vi "read_config_file.vi"(8 "error in (no error)":errorcluster caption="错误输入（无错误）") -> (0 "error out":errorcluster caption="错误输出")   [LabVIEW 2015]
uses:
  globals/global_configuration_options.vi
  globals/global_device_tree_items.vi
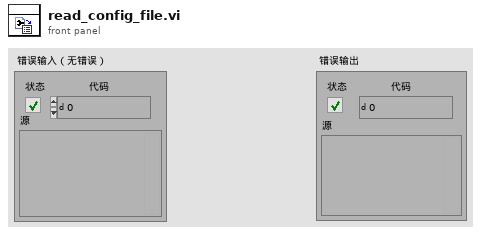
[diagram p1: front panel]
types:
  T1 = cluster{"Left Cell String":string, "Child Text":string[], "Child Tag":string, "Item Indent":i32, "Child Only?":bool, "Glyph Index":i32}[]
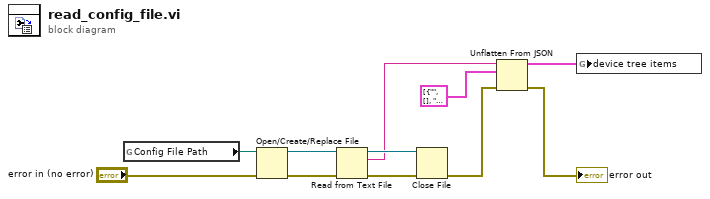
[diagram p0: block diagram]
diagram:
  n1 = global read "global_configuration_options.vi" "Config File Path"() -> (w11:path)
  n2 = Open/Create/Replace File(file path (use dialog)=w11, error in="error in (no error)") -> (refnum out=w9:refnum<file>, error out=w8:errorcluster)  [unwired: 4 in, 1 out]
  n3 = Read from Text File(file (use dialog)=w9, error in=w8) -> (refnum out=w7:refnum<file>, text=w5:string, error out=w6:errorcluster)  [unwired: 2 in, 1 out]
  n4 = Close File(refnum=w7, error in=w6) -> (error out=w4:errorcluster)  [unwired: 1 out]
  n5 = Unflatten From JSON(JSON string=w5, type and defaults=T1 [{"Left Cell String"="", "Child Text"=[], "Child Tag"="", "Item Indent"=0, "Child Only?"=FALSE, "Glyph Index"=1}, {"Left Cell String"="Mod1 (Slot1 NI 9239)", "Child Text"=[], "Child Tag"="Mod1", "Item Indent"=1, "Child Only?"=FALSE, "Glyph Index"=3}, {"Left Cell String"="FCXF-X-02-A01", "Child Text"=[], "Child Tag"="FCXF-X-02-A01", "Item Indent"=2, "Child Only?"=TRUE, "Glyph Index"=4}, {"Left Cell String"="FCXF-X-03-A01", "Child Text"=[], "Child Tag"="FCXF-X-03-A01", "Item Indent"=2, "Child Only?"=TRUE, "Glyph Index"=4}, {"Left Cell String"="FCXF-X-03-A02", "Child Text"=[], "Child Tag"="FCXF-X-03-A02", "Item Indent"=2, "Child Only?"=TRUE, "Glyph Index"=4}, {"Left Cell String"="FCXF-X-04-A01", "Child Text"=[], "Child Tag"="FCXF-X-04-A01", "Item Indent"=2, "Child Only?"=TRUE, "Glyph Index"=4}, {"Left Cell String"="Mod2 (Slot2 NI 9219)", "Child Text"=[], "Child Tag"="Mod2", "Item Indent"=1, "Child Only?"=FALSE, "Glyph Index"=3}, {"Left Cell String"="FCXF-X-02-S01", "Child Text"=[], "Child Tag"="FCXF-X-02-S01", "Item Indent"=2, "Child Only?"=TRUE, "Glyph Index"=4}, {"Left Cell String"="FCXF-X-02-S02", "Child Text"=[], "Child Tag"="FCXF-X-02-S02", "Item Indent"=2, "Child Only?"=TRUE, "Glyph Index"=4}, {"Left Cell String"="FCXF-X-02-S03", "Child Text"=[], "Child Tag"="FCXF-X-02-S03", "Item Indent"=2, "Child Only?"=TRUE, "Glyph Index"=4}, {"Left Cell String"="FCXF-X-02-S04", "Child Text"=[], "Child Tag"="FCXF-X-02-S04", "Item Indent"=2, "Child Only?"=TRUE, "Glyph Index"=4}, {"Left Cell String"="Mod4 (Slot4 NI 9219)", "Child Text"=[], "Child Tag"="Mod4", "Item Indent"=1, "Child Only?"=FALSE, "Glyph Index"=3}, {"Left Cell String"="FCXF-X-03-S01", "Child Text"=[], "Child Tag"="FCXF-X-03-S01", "Item Indent"=2, "Child Only?"=TRUE, "Glyph Index"=4}, {"Left Cell String"="FCXF-X-03-S02", "Child Text"=[], "Child Tag"="FCXF-X-03-S02", "Item Indent"=2, "Child Only?"=TRUE, "Glyph Index"=4}, {"Left Cell String"="FCXF-X-03-S03", "Child Text"=[], "Child Tag"="FCXF-X-03-S03", "Item Indent"=2, "Child Only?"=TRUE, "Glyph Index"=4}, {"Left Cell String"="FCXF-X-03-S04", "Child Text"=[], "Child Tag"="FCXF-X-03-S04", "Item Indent"=2, "Child Only?"=TRUE, "Glyph Index"=4}, {"Left Cell String"="Mod6 (Slot6 NI 9219)", "Child Text"=[], "Child Tag"="Mod6", "Item Indent"=1, "Child Only?"=FALSE, "Glyph Index"=3}, {"Left Cell String"="FCXF-X-03-S05", "Child Text"=[], "Child Tag"="FCXF-X-03-S05", "Item Indent"=2, "Child Only?"=TRUE, "Glyph Index"=4}, {"Left Cell String"="FCXF-X-03-S06", "Child Text"=[], "Child Tag"="FCXF-X-03-S06", "Item Indent"=2, "Child Only?"=TRUE, "Glyph Index"=4}, {"Left Cell String"="Mod8 (Slot8 NI 9219)", "Child Text"=[], "Child Tag"="Mod8", "Item Indent"=1, "Child Only?"=FALSE, "Glyph Index"=3}, {"Left Cell String"="FCXF-X-04-S01", "Child Text"=[], "Child Tag"="FCXF-X-04-S01", "Item Indent"=2, "Child Only?"=TRUE, "Glyph Index"=4}, {"Left Cell String"="FCXF-X-04-S02", "Child Text"=[], "Child Tag"="FCXF-X-04-S02", "Item Indent"=2, "Child Only?"=TRUE, "Glyph Index"=4}, {"Left Cell String"="FCXF-X-04-S03", "Child Text"=[], "Child Tag"="FCXF-X-04-S03", "Item Indent"=2, "Child Only?"=TRUE, "Glyph Index"=4}, {"Left Cell String"="FCXF-X-04-S04", "Child Text"=[], "Child Tag"="FCXF-X-04-S04", "Item Indent"=2, "Child Only?"=TRUE, "Glyph Index"=4}, {"Left Cell String"="Mod9 (USB1 ICPCON 7005)", "Child Text"=[], "Child Tag"="Mod9", "Item Indent"=1, "Child Only?"=FALSE, "Glyph Index"=3}, {"Left Cell String"="FCXF-X-02-T01", "Child Text"=[], "Child Tag"="FCXF-X-02-T01", "Item Indent"=2, "Child Only?"=TRUE, "Glyph Index"=4}, {"Left Cell String"="FCXF-X-02-T02", "Child Text"=[], "Child Tag"="FCXF-X-02-T02", "Item Indent"=2, "Child Only?"=TRUE, "Glyph Index"=4}, {"Left Cell String"="FCXF-X-02-T03", "Child Text"=[], "Child Tag"="FCXF-X-02-T03", "Item Indent"=2, "Child Only?"=TRUE, "Glyph Index"=4}, {"Left Cell String"="FCXF-X-02-T04", "Child Text"=[], "Child Tag"="FCXF-X-02-T04", "Item Indent"=2, "Child Only?"=TRUE, "Glyph Index"=4}, {"Left Cell String"="FCXF-X-03-T01", "Child Text"=[], "Child Tag"="FCXF-X-03-T01", "Item Indent"=2, "Child Only?"=TRUE, "Glyph Index"=4}, {"Left Cell String"="FCXF-X-03-T02", "Child Text"=[], "Child Tag"="FCXF-X-03-T02", "Item Indent"=2, "Child Only?"=TRUE, "Glyph Index"=4}, {"Left Cell String"="FCXF-X-03-T03", "Child Text"=[], "Child Tag"="FCXF-X-03-T03", "Item Indent"=2, "Child Only?"=TRUE, "Glyph Index"=4}, {"Left Cell String"="Mod10 (USB1 ICPCON 7005)", "Child Text"=[], "Child Tag"="Mod10", "Item Indent"=1, "Child Only?"=FALSE, "Glyph Index"=3}, {"Left Cell String"="FCXF-X-03-T04", "Child Text"=[], "Child Tag"="FCXF-X-03-T04", "Item Indent"=2, "Child Only?"=TRUE, "Glyph Index"=4}, {"Left Cell String"="FCXF-X-03-T05", "Child Text"=[], "Child Tag"="FCXF-X-03-T05", "Item Indent"=2, "Child Only?"=TRUE, "Glyph Index"=4}, {"Left Cell String"="FCXF-X-03-T06", "Child Text"=[], "Child Tag"="FCXF-X-03-T06", "Item Indent"=2, "Child Only?"=TRUE, "Glyph Index"=4}, {"Left Cell String"="FCXF-X-04-T01", "Child Text"=[], "Child Tag"="FCXF-X-04-T01", "Item Indent"=2, "Child Only?"=TRUE, "Glyph Index"=4}, {"Left Cell String"="FCXF-X-04-T02", "Child Text"=[], "Child Tag"="FCXF-X-04-T02", "Item Indent"=2, "Child Only?"=TRUE, "Glyph Index"=4}, {"Left Cell String"="FCXF-X-04-T03", "Child Text"=[], "Child Tag"="FCXF-X-04-T03", "Item Indent"=2, "Child Only?"=TRUE, "Glyph Index"=4}, {"Left Cell String"="FCXF-X-04-T04", "Child Text"=[], "Child Tag"="FCXF-X-04-T04", "Item Indent"=2, "Child Only?"=TRUE, "Glyph Index"=4}] ("device tree items"), error in (no error)=w4) -> (value=w1:T1, error out=→"error out":errorcluster)  [unwired: 4 in]
  n6 = global write "global_device_tree_items.vi" "device tree items"(w1) -> ()
